vi "Auto Nbr. STEP.vi"(8 "error in (no error)":errorcluster, 9 "index (col)":i32, 10 "STEP in":refnum<class "STEP.lvclass">, 11 "All Sequence STEPs in":refnum<class "STEP.lvclass">[](array[class])) -> (0 "error out":errorcluster, 1 "Discarded?":bool, 3 "All Sequence STEPs out":refnum<class "STEP.lvclass">[](array[class]))   [LabVIEW 2014, in "SeqLoop.lvlib"]
uses:
  SeqLoop.lvlib
  Classes/STEP/STEP.lvclass
  Classes/STEP/STEP.lvclass/STEP.ctl
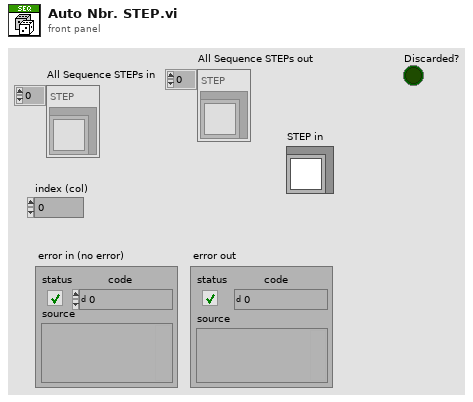
[diagram p1: front panel]
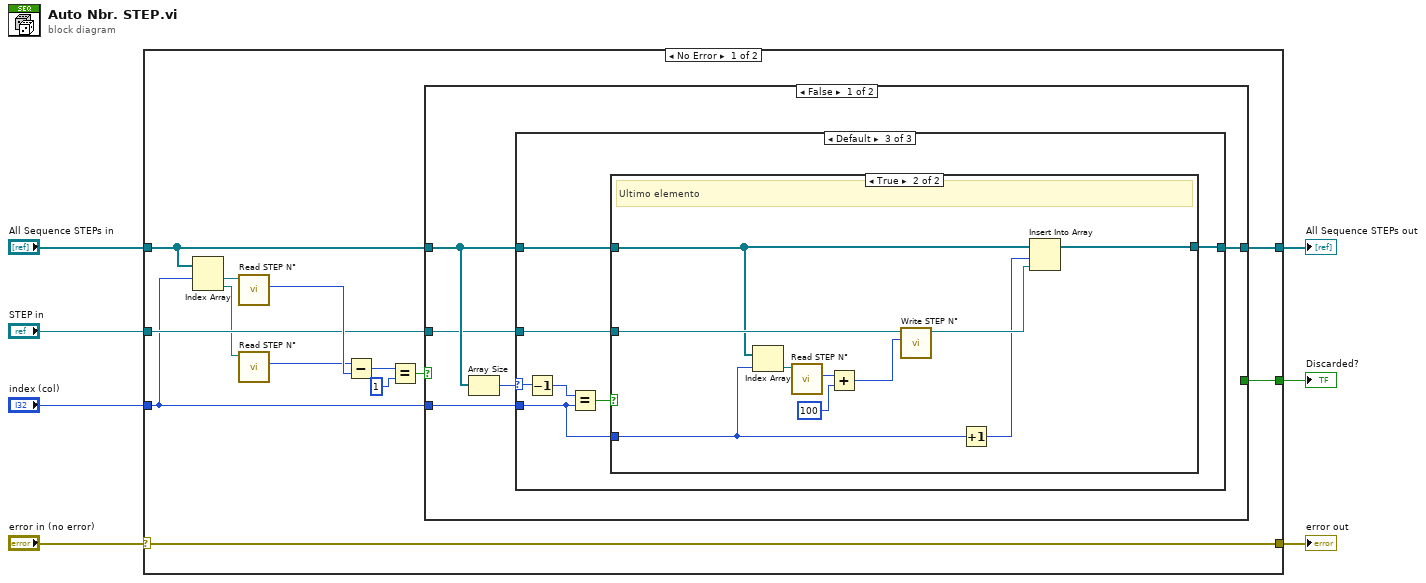
[diagram p0: block diagram]
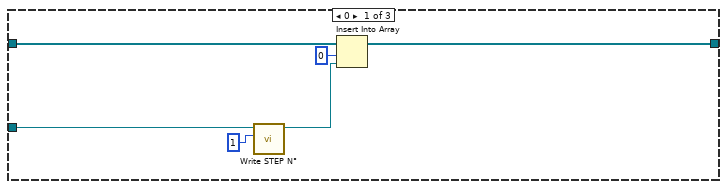
[diagram p2: hidden frame]
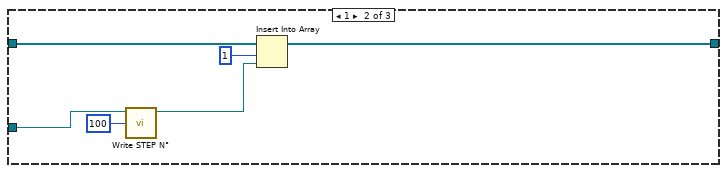
[diagram p3: hidden frame]
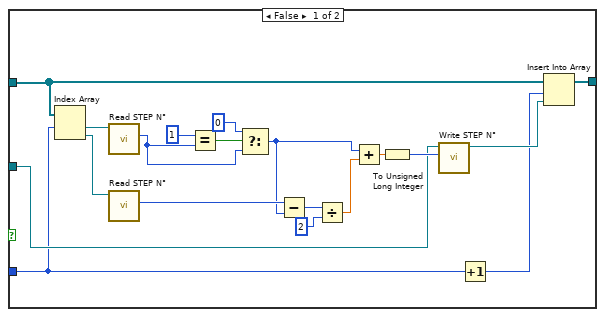
[diagram p4: hidden frame]
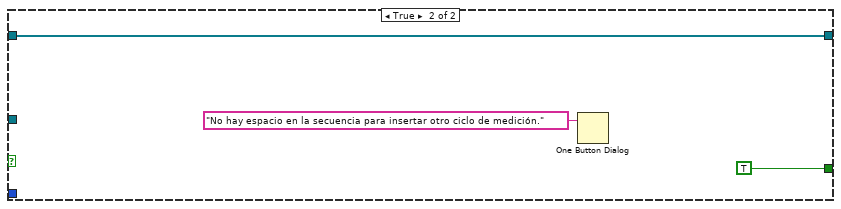
[diagram p5: hidden frame]
diagram:
  n1 = case shown="No Error" "error in (no error)" {
    selector: "error in (no error)" -> [w20 w78]
    tunnel: "All Sequence STEPs in" -> [w18 w77]
    tunnel: "index (col)" -> [w8 _]
    tunnel: [w20 w78] -> w4
    tunnel: "STEP in" -> [w12 _]
    tunnel: [w19 w77] -> w2
    tunnel: [w9 _] -> w1
    frame No Error {
      n2 = Index Array(array=w18, index #1=w8) -> (element #1=w11:refnum<class "STEP.lvclass">, element #2=w10:refnum<class "STEP.lvclass">)  [unwired: 1 in]
      n3 = call "Read STEP N°.vi"("STEP in"=w11) -> ("STEP N°"=w17:u32)  [unwired: 9 in, 1 out]
      n4 = call "Read STEP N°.vi"("STEP in"=w10) -> ("STEP N°"=w16:u32)  [unwired: 9 in, 1 out]
      n5 = Subtract(x=w16, y=w17) -> (x-y=w14:u32)
      n6 = Equal?(x=w14, y=u32 1) -> (x = y?=w15:bool)
      n7 = case shown="False" w15 {
        tunnel: [w24 w76] -> w19
        tunnel: w18 -> [w23 w76]
        tunnel: w8 -> [w22 _]
        tunnel: w12 -> [w21 _]
        tunnel: [_ TRUE] -> w9
        frame False {
          n8 = Array Size(array=w23) -> (size(s)=w25:i32)
          n9 = case shown="Default" w25 {
            selector: w25 -> [_ _ w44]
            tunnel: w23 -> [w29 w36 w40]
            tunnel: w22 -> [_ _ w39]
            tunnel: w21 -> [w30 w32 w41]
            tunnel: [w27 w33 w38] -> w24
            frame 0 {
              n10 = call "Write STEP N°.vi"("STEP N°"=u32 1, "STEP in"=w30) -> ("STEP out"=w28:refnum<class "STEP.lvclass">)  [unwired: 8 in, 1 out]
              n11 = Insert Into Array(array=w29, index=0, new element=w28) -> (w27:refnum<class "STEP.lvclass">[])
            }
            frame 1 {
              n12 = call "Write STEP N°.vi"("STEP N°"=u32 100, "STEP in"=w32) -> ("STEP out"=w35:refnum<class "STEP.lvclass">)  [unwired: 8 in, 1 out]
              n13 = Insert Into Array(array=w36, index=1, new element=w35) -> (w33:refnum<class "STEP.lvclass">[])
            }
            frame Default {
              n14 = Decrement(x=w44) -> (x-1=w43:i32)
              n15 = Equal?(x=w43, y=w39) -> (x = y?=w42:bool)
              n16 = case shown="True" w42 {
                tunnel: w41 -> [w50 w73]
                tunnel: w40 -> [w48 w68]
                tunnel: w39 -> [w45 w65]
                tunnel: [w49 w67] -> w38
                frame False {
                  n17 = Index Array(array=w48, index #1=w45) -> (element #1=w63:refnum<class "STEP.lvclass">, element #2=w62:refnum<class "STEP.lvclass">)  [unwired: 1 in]
                  n18 = call "Read STEP N°.vi"("STEP in"=w63) -> ("STEP N°"=w55:u32)  [unwired: 9 in, 1 out]
                  n19 = call "Read STEP N°.vi"("STEP in"=w62) -> ("STEP N°"=w58:u32)  [unwired: 9 in, 1 out]
                  n20 = Equal?(x=u32 1 ("y"), y=w55) -> (x = y?=w60:bool)
                  n21 = Select(t=u32 0 ("y"), s=w60, f=w55) -> (s? t:f=w54:u32)
                  n22 = Subtract(x=w58, y=w54) -> (x-y=w57:u32)
                  n23 = Divide(x=w57, y=u32 2) -> (x/y=w53:dbl)
                  n24 = Add(x=w54, y=w53) -> (x+y=w52:dbl)
                  n25 = To Unsigned Long Integer(number=w52) -> (unsigned 32bit integer=w51:u32)
                  n26 = call "Write STEP N°.vi"("STEP N°"=w51, "STEP in"=w50) -> ("STEP out"=w47:refnum<class "STEP.lvclass">)  [unwired: 8 in, 1 out]
                  n27 = Increment(x=w45) -> (x+1=w46:i32)
                  n28 = Insert Into Array(array=w48, index=w46, new element=w47) -> (w49:refnum<class "STEP.lvclass">[])
                }
                frame True {
                  # "Ultimo elemento"
                  n29 = Index Array(array=w68, index=w65) -> (element=w72:refnum<class "STEP.lvclass">)
                  n30 = call "Read STEP N°.vi"("STEP in"=w72) -> ("STEP N°"=w70:u32)  [unwired: 9 in, 1 out]
                  n31 = Add(x=w70, y=u32 100) -> (x+y=w71:u32)
                  n32 = call "Write STEP N°.vi"("STEP N°"=w71, "STEP in"=w73) -> ("STEP out"=w66:refnum<class "STEP.lvclass">)  [unwired: 8 in, 1 out]
                  n33 = Increment(x=w65) -> (x+1=w64:i32)
                  n34 = Insert Into Array(array=w68, index=w64, new element=w66) -> (w67:refnum<class "STEP.lvclass">[])
                }
              }
            }
          }
        }
        frame True {
          n35 = One Button Dialog(message="No hay espacio en la secuencia para insertar otro ciclo de medición.") -> ()  [unwired: 1 in, 1 out]
        }
      }
    }
    frame Error {
    }
  }
  "error out" <- w4
  "All Sequence STEPs out" <- w2
  "Discarded?" <- w1
